vi "Pre Launch Init.vi"(11 "Splash Screen Contract Model in":refnum<class "Splash Screen Contract Model.lvclass">) -> (0 "error out":errorcluster, 3 "Splash Screen Contract Model out":refnum<class "Splash Screen Contract Model.lvclass">)   [LabVIEW 2019, in "Splash Screen Contract Model.lvclass"]
doc: "(<B>Filename</B>: Actor Framework.lvlib:Actor.lvclass:Pre Launch Init.vi)\n\nDefines behavior that occurs after the Launch Nested Actor method is invoked but before the actor's Actor Core method begins running.\n\nBy default, this method does nothing. A descendant class may override it to define behavior."
uses:
  <vilib>/gpm_packages/@cs/Car-wash/Source/Splash Screen Contract Model/Splash Screen Contract Model.lvclass
  C:/Program Files/National Instruments/LabVIEW 2019/vi.lib/ActorFramework/Actor/Actor.lvclass
  <vilib>/ActorFramework/Actor/Actor.lvclass/Actor.ctl
  <vilib>/ActorFramework/Message Enqueuer/Message Enqueuer.lvclass/Message Enqueuer.ctl
  <vilib>/ActorFramework/Message Enqueuer/Enqueue.vi
  <vilib>/ActorFramework/Message Enqueuer/Init from Existing Queue.vi
  <vilib>/gpm_packages/@cs/Car-wash/Source/Splash Screen Contract Model Messages/Create Time Delayed Send Message Msg/Create Time Delayed Send Message Msg.lvclass
  C:/Program Files/National Instruments/LabVIEW 2019/vi.lib/ActorFramework/Message/Message.lvclass
  <vilib>/ActorFramework/Message Priority Queue/Priority Enqueue.vi
  <vilib>/gpm_packages/@cs/Car-wash/Source/iSplash Screen Contract Model/iSplash Screen Contract Model.lvclass
  <vilib>/ActorFramework/Message Enqueuer/Message Enqueuer.lvclass
  <vilib>/ActorFramework/Actor/Actor.lvclass
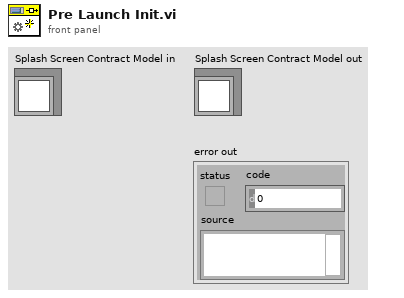
[diagram p1: front panel]
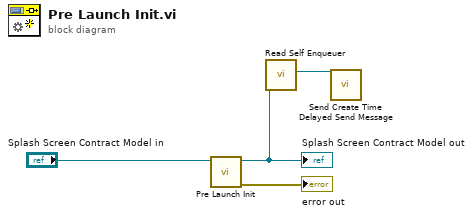
[diagram p0: block diagram]
diagram:
  n1 = call-parent "Pre Launch Init.vi"("IModel in"="Splash Screen Contract Model in") -> ("error out"=→"error out":errorcluster, "IModel out"=w2:refnum<class "Splash Screen Contract Model.lvclass">)  [unwired: 9 in]
  "Splash Screen Contract Model out" <- w2
  n2 = call <vilib>:"Read Self Enqueuer.vi"("Actor"=w2) -> ("Self Enqueuer"=w1:refnum<class "Message Enqueuer.lvclass">)  [unwired: 10 in]
  n3 = call <vilib>:"Send Create Time Delayed Send Message.vi"("Message Enqueuer"=w1) -> ()  [unwired: 9 in, 2 out]
